vi "Bid farewell.vi"(8 "error in (no error)":errorcluster, 11 "Guardian in":refnum<class "Guardian.lvclass">) -> (0 "error out":errorcluster, 3 "Guardian out":refnum<class "Guardian.lvclass">)   [LabVIEW 2026, in "TALOS.lvlib" / "Guardian.lvlib" / "Guardian.lvclass"]
uses:
  Guardian.lvclass
  C:/LabVIEW Code/TALOS/talos/Ancestor/Ancestor/Ancestor.lvclass
  Ancestor/Ancestor/Ancestor.lvclass/Ancestor.ctl
  Guardian.lvclass/Guardian.ctl
  Classes/Guardian List/Guardian List.lvclass
  builds/Actor Framework PPL/Actor Framework.lvlibp/1abvi3w/vi.lib/ActorFramework/Message Enqueuer/Message Priority.ctl
  builds/Actor Framework PPL/Actor Framework.lvlibp/1abvi3w/vi.lib/ActorFramework/Message Enqueuer/Message Enqueuer.lvclass
  TALOS.lvlib
  Ancestor/Ancestor/Ancestor.lvclass
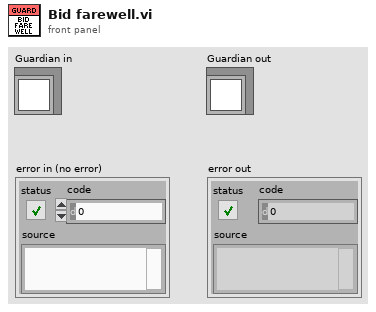
[diagram p1: front panel]
types:
  T1 = typedef "Actor Framework.lvlibp/Message Enqueuer.lvclass/Message Priority.ctl" = enum16{"Low", "Normal", "High"}
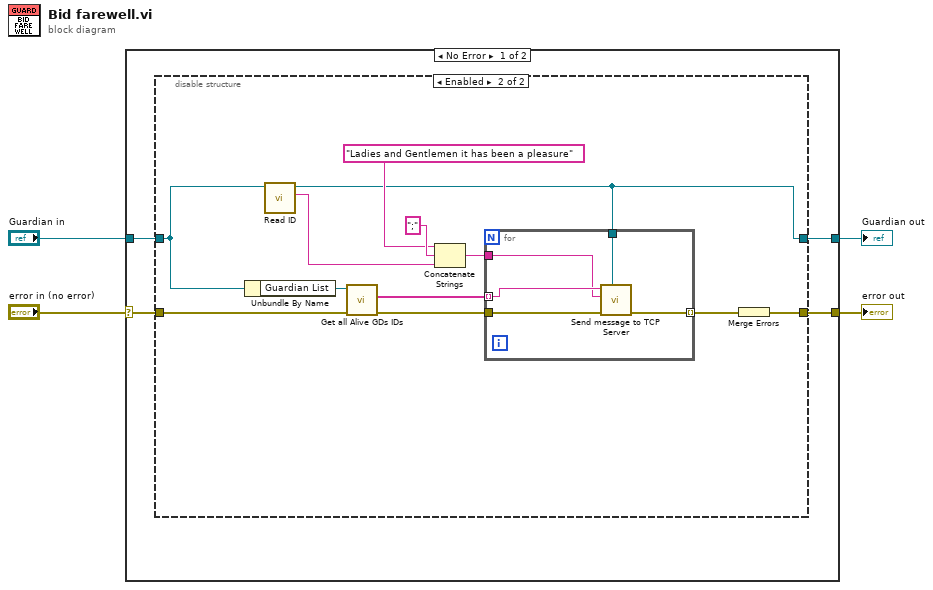
[diagram p0: block diagram]
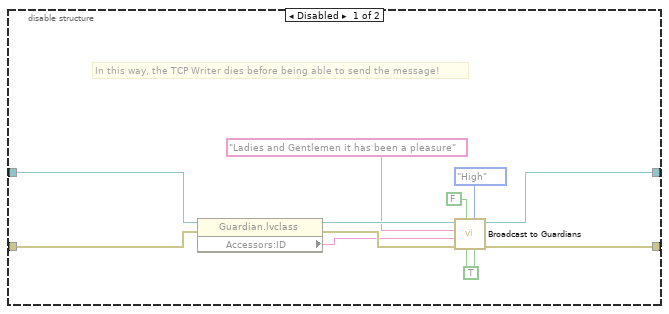
[diagram p2: hidden frame]
diagram:
  n1 = case shown="No Error" "error in (no error)" {
    selector: "error in (no error)" -> [w8 w37]
    tunnel: "Guardian in" -> [w7 w38]
    tunnel: [w6 w37] -> w2
    tunnel: [w5 w38] -> w1
    frame No Error {
      n2 = disable-structure shown="Enabled" {
        disable-tunnel: w8 -> [w18 w21]
        disable-tunnel: w7 -> [w15 w20]
        disable-tunnel: [w10 w27] -> w6
        disable-tunnel: [w9 w25] -> w5
        frame Disabled {
          w13 = TRUE ("Critical PCs also?")
          # "In this way, the TCP Writer dies before being able to send the message!"
          n3 = property class="Guardian.lvclass"(reference=w15, error in=w18) -> (reference out=w16:refnum<class "Guardian.lvclass">, error out=w19:errorcluster, "Accessors:ID"=w17:string)
          n4 = call "Broadcast to Guardians.vi"("Critical PCs also?"=w13, "Message Priority"=Message_Priority."High", "Only active ones?"=w13, "Local also?"=FALSE, "error in (no error)"=w19, "Data"=w17, "Message"="Ladies and Gentlemen it has been a pleasure", "Guardian in"=w16) -> ("error out"=w10:errorcluster, "Guardian out"=w9:refnum<class "Guardian.lvclass">)  [unwired: 2 in]
        }
        frame Enabled {
          n5 = Unbundle By Name(w20) -> ("Guardian List"=w24:refnum<class "Guardian List.lvclass">)
          n6 = call "Read ID.vi"("Ancestor in"=w20) -> ("ID"=w31:string, "Ancestor out"=w25:refnum<class "Guardian.lvclass">)  [unwired: 8 in, 1 out]
          n7 = call-dynamic "Get all Alive GDs IDs.vi"("error in (no error)"=w21, "Guardian List in"=w24) -> ("error out"=w22:errorcluster, "Alive GDs IDs"=w23:string[])  [unwired: 7 in, 1 out]
          n8 = Concatenate Strings("Ladies and Gentlemen it has been a pleasure" ("Message"), ";" ("string"), w31) -> (w29:string)
          n9 = for {
            tunnel: w22 -> [w36]
            tunnel: [w32] -> w28 mode=indexing
            tunnel: w23 -> [w35] mode=indexing
            tunnel: w29 -> [w33]
            tunnel: w25 -> [w34]
            n10 = call "Send message to TCP Server.vi"("LabVIEW Object"=w34, "error in (no error)"=w36, "String"=w33, "Guardian ID"=w35) -> ("error out"=w32:errorcluster)  [unwired: 7 in]
          }
          n11 = Merge Errors(w28) -> (w27:errorcluster)
        }
      }
    }
    frame Error {
    }
  }
  "error out" <- w2
  "Guardian out" <- w1
